vi "getWaypoints.vi"(8 "Error In":errorcluster, 11 "PassBouy in":refnum<class "PassBouy.lvclass">) -> (0 "Error Out":errorcluster, 2 "Waypoint Array":refnum<class "Waypoint.lvclass">[](array[class]), 3 "PassBouy out":refnum<class "PassBouy.lvclass">)   [LabVIEW 2013, in "PassBouy.lvclass"]
uses:
  PassBouy.lvclass
  trunk/Software/2-Think/2 Classes/Missions/GenericMission/GenericMission.lvclass
  Waypoint/Waypoint.lvclass
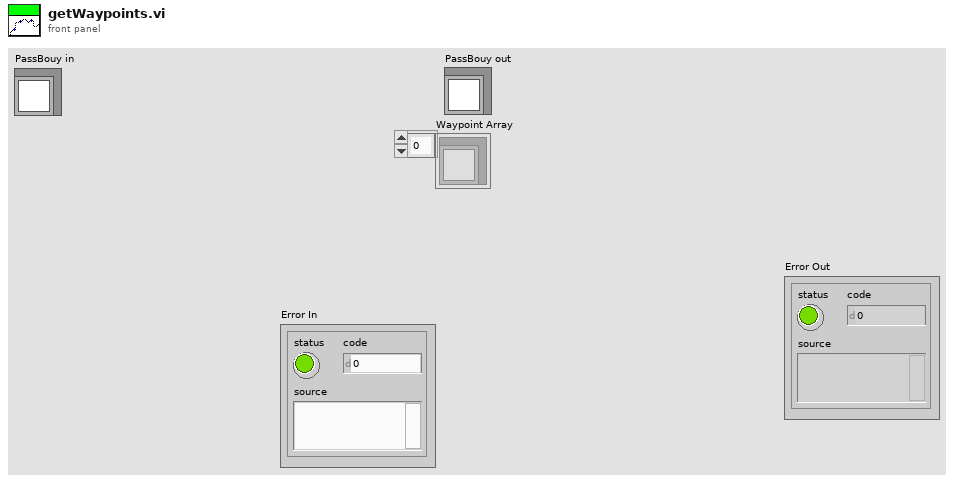
[diagram p1: front panel]
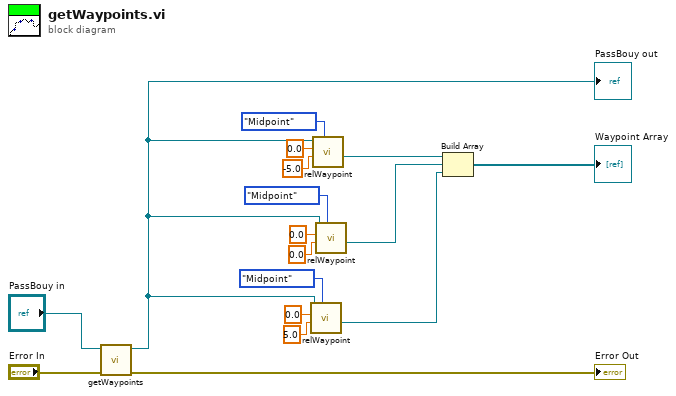
[diagram p0: block diagram]
diagram:
  n1 = call-parent "getWaypoints.vi"("Error In"="Error In", "GenericMission in"="PassBouy in") -> ("Error Out"=→"Error Out":errorcluster, "GenericMission out"=w1:refnum<class "PassBouy.lvclass">)  [unwired: 7 in, 1 out]
  "PassBouy out" <- w1
  n2 = call "relWaypoint.vi"("Base Point"=enum16{"Port", "Midpoint", "Starboard"}."Midpoint", "Y coord"=5.0 ("X coord"), "X coord"=0.0, "PassBouy.lvclass"=w1) -> ("Waypoint Out"=w4:refnum<class "Waypoint.lvclass">)  [unwired: 5 in, 2 out]
  n3 = call "relWaypoint.vi"("Base Point"=enum16{"Port", "Midpoint", "Starboard"}."Midpoint", "Y coord"=-5.0 ("X coord"), "X coord"=0.0, "PassBouy.lvclass"=w1) -> ("Waypoint Out"=w13:refnum<class "Waypoint.lvclass">)  [unwired: 5 in, 2 out]
  n4 = call "relWaypoint.vi"("Base Point"=enum16{"Port", "Midpoint", "Starboard"}."Midpoint", "Y coord"=0.0 ("X coord"), "X coord"=0.0, "PassBouy.lvclass"=w1) -> ("Waypoint Out"=w3:refnum<class "Waypoint.lvclass">)  [unwired: 5 in, 2 out]
  n5 = Build Array(w13, w3, w4) -> (→"Waypoint Array":refnum<class "Waypoint.lvclass">[])
